vi "Vector3DScale.vi"(9 "Scale Factor":dbl, 10 "Vector3D":T1) -> (2 "Scaled Vector":T1)   [LabVIEW 2018]
uses:
  Vector3D.ctl
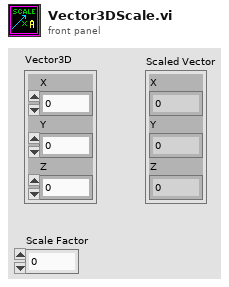
[diagram p1: front panel]
types:
  T1 = typedef "Vector3D.ctl" = cluster{"X":dbl, "Y":dbl, "Z":dbl}
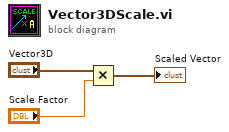
[diagram p0: block diagram]
diagram:
  n1 = Multiply(x="Vector3D", y="Scale Factor") -> (x*y=→"Scaled Vector":T1)
